vi "Set Default.vi"(11 "String in":refnum<class "String.lvclass">) -> (3 "String out":refnum<class "String.lvclass">)   [LabVIEW 2020, in "Conditum.lvlib" / "Columns.lvlib" / "String.lvclass"]
uses:
  String.lvclass
  Type/Type.lvclass
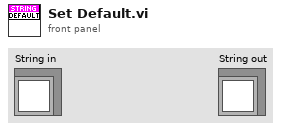
[diagram p1: front panel]
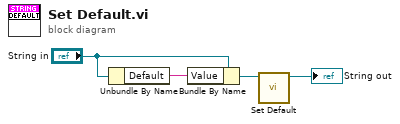
[diagram p0: block diagram]
diagram:
  n1 = Unbundle By Name("String in") -> ("Default"=w4:string)
  n2 = Bundle By Name(cluster="String in", "Value"=w4) -> (w3:refnum<class "String.lvclass">)
  n3 = call-parent "Set Default.vi"("Type in"=w3) -> ("Type out"=→"String out":refnum<class "String.lvclass">)  [unwired: 10 in]
